vi "PH_SSAC.evt call set dt Gauss smooth.vi"(0 "i ref in":refnum<vi>, 1 "Instance":string, 2 "dt (Gauss smooth)":dbl, 5 "error in":errorcluster) -> (14 "i ref out":refnum<vi>, 19 "error out":errorcluster)   [LabVIEW 2014, in "PH_SSAC.lvlib"]
doc: "This VI calls an event case by a simple call."
uses:
  PH_SSAC.lvlib
  CSCore/CSSystem/CoreLib/CoreLib.double 2 byte array.vi
  CSCore/CSSystem/CoreLib/CoreLib.lvlib
  CSCore/BaseProcess/BaseProcess.lvlib
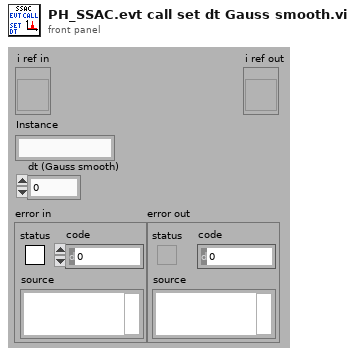
[diagram p1: front panel]
types:
  T1 = typedef "CoreDefs.rawDataType.ctl" = i8[]
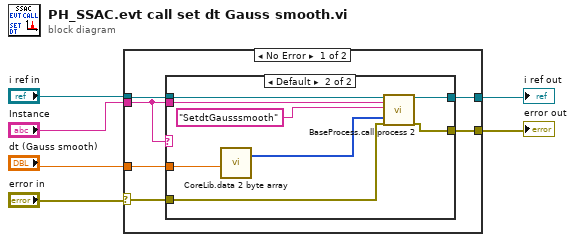
[diagram p0: block diagram]
diagram:
  n1 = case shown="No Error" "error in" {
    selector: "error in" -> [w9 w23]
    tunnel: [w12 w24] -> w4
    tunnel: [w11 w23] -> w3
    tunnel: "i ref in" -> [w10 w24]
    tunnel: "Instance" -> [w8 _]
    tunnel: "dt (Gauss smooth)" -> [w7 _]
    frame No Error {
      n2 = case shown="Default" w8 {
        tunnel: [w14 w21] -> w12
        tunnel: [w13 w20] -> w11
        tunnel: w10 -> [w14 w19]
        tunnel: w8 -> [_ w18]
        tunnel: w9 -> [w13 w17]
        tunnel: w7 -> [_ w15]
        frame "N/A" {
        }
        frame Default {
          n3 = call-poly "CoreLib.data 2 byte array.vi"("f64"=w15) -> ("byteArray out"=w16:T1)  [unwired: 18 in]
          n4 = call "BaseProcess.call process 2.vi"("i ref in"=w19, "Object"=w18, "Selector"="SetdtGausssmooth", "Data"=w16, "error in (no error)"=w17) -> ("i ref out"=w21:refnum<vi>, "error out"=w20:errorcluster)  [unwired: 13 in]
        }
      }
    }
    frame Error {
    }
  }
  "i ref out" <- w4
  "error out" <- w3
